vi "Example.vi"   [LabVIEW 2018]
uses:
  src/MPU.lvclass
  <vilib>/rvi/DataTransferAndStorage/Container/Common/niFpgaContainerGetUniqueNameForEmu.vi
  <vilib>/rvi/DataTransferAndStorage/Container/Common/niFpgaContainerSetEmuInfo.vi
  <vilib>/rvi/eio/common/nirviEmuReportErrorAndStop.vi
  <vilib>/rvi/LocalResourceManager/LocalResourceManager.xnode
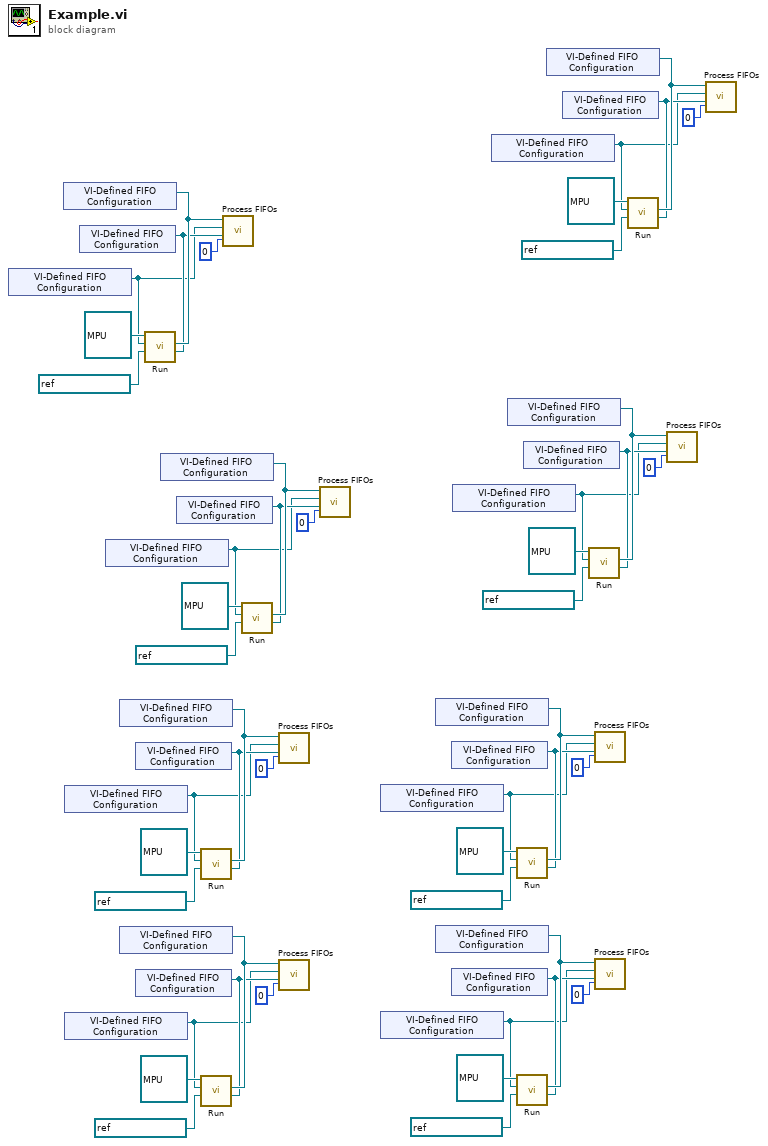
[diagram p0: block diagram]
diagram:
  n1 = xnode "VI-Defined FIFO Configuration"() -> ("FIFO Out"=w43:refnum<k21>)
  n2 = xnode "VI-Defined FIFO Configuration"() -> ("FIFO Out"=w46:refnum<k21>)
  n3 = xnode "VI-Defined FIFO Configuration"() -> ("FIFO Out"=w19:refnum<k21>)
  n4 = xnode "VI-Defined FIFO Configuration"() -> ("FIFO Out"=w7:refnum<k21>)
  n5 = xnode "VI-Defined FIFO Configuration"() -> ("FIFO Out"=w45:refnum<k21>)
  n6 = xnode "VI-Defined FIFO Configuration"() -> ("FIFO Out"=w31:refnum<k21>)
  n7 = xnode "VI-Defined FIFO Configuration"() -> ("FIFO Out"=w22:refnum<k21>)
  n8 = xnode "VI-Defined FIFO Configuration"() -> ("FIFO Out"=w10:refnum<k21>)
  n9 = xnode "VI-Defined FIFO Configuration"() -> ("FIFO Out"=w21:refnum<k21>)
  n10 = xnode "VI-Defined FIFO Configuration"() -> ("FIFO Out"=w9:refnum<k21>)
  n11 = call-dynamic "Run.vi"("DebugOut"=w45, "Telemetry"=w46, "Port"=refnum<k21> "Mod1\\Port1", "Command FIFO"=w43, "MPU in"=refnum<class "MPU.lvclass"> refnum ("Modbus_Processing_Unit.lvlib:MPU.lvclass")) -> ()  [unwired: 4 in, 2 out]
  n12 = xnode "VI-Defined FIFO Configuration"() -> ("FIFO Out"=w34:refnum<k21>)
  n13 = xnode "VI-Defined FIFO Configuration"() -> ("FIFO Out"=w33:refnum<k21>)
  n14 = call-dynamic "Run.vi"("DebugOut"=w21, "Telemetry"=w22, "Port"=refnum<k21> "Mod1\\Port3", "Command FIFO"=w19, "MPU in"=refnum<class "MPU.lvclass"> refnum ("Modbus_Processing_Unit.lvlib:MPU.lvclass")) -> ()  [unwired: 4 in, 2 out]
  n15 = call-dynamic "Run.vi"("DebugOut"=w9, "Telemetry"=w10, "Port"=refnum<k21> "Mod1\\Port4", "Command FIFO"=w7, "MPU in"=refnum<class "MPU.lvclass"> refnum ("Modbus_Processing_Unit.lvlib:MPU.lvclass")) -> ()  [unwired: 4 in, 2 out]
  n16 = call "Process FIFOs.vi"("Timeout"=0, "FIFO Out 2"=w45, "FIFO Out"=w43, "Refnum in"=w46) -> ()  [unwired: 7 in, 1 out]
  n17 = call-dynamic "Run.vi"("DebugOut"=w33, "Telemetry"=w34, "Port"=refnum<k21> "Mod1\\Port2", "Command FIFO"=w31, "MPU in"=refnum<class "MPU.lvclass"> refnum ("Modbus_Processing_Unit.lvlib:MPU.lvclass")) -> ()  [unwired: 4 in, 2 out]
  n18 = call "Process FIFOs.vi"("Timeout"=0, "FIFO Out 2"=w21, "FIFO Out"=w19, "Refnum in"=w22) -> ()  [unwired: 7 in, 1 out]
  n19 = call "Process FIFOs.vi"("Timeout"=0, "FIFO Out 2"=w9, "FIFO Out"=w7, "Refnum in"=w10) -> ()  [unwired: 7 in, 1 out]
  n20 = call "Process FIFOs.vi"("Timeout"=0, "FIFO Out 2"=w33, "FIFO Out"=w31, "Refnum in"=w34) -> ()  [unwired: 7 in, 1 out]
  n21 = xnode "VI-Defined FIFO Configuration"() -> ("FIFO Out"=w13:refnum<k21>)
  n22 = xnode "VI-Defined FIFO Configuration"() -> ("FIFO Out"=w1:refnum<k21>)
  n23 = xnode "VI-Defined FIFO Configuration"() -> ("FIFO Out"=w16:refnum<k21>)
  n24 = xnode "VI-Defined FIFO Configuration"() -> ("FIFO Out"=w4:refnum<k21>)
  n25 = xnode "VI-Defined FIFO Configuration"() -> ("FIFO Out"=w15:refnum<k21>)
  n26 = xnode "VI-Defined FIFO Configuration"() -> ("FIFO Out"=w3:refnum<k21>)
  n27 = xnode "VI-Defined FIFO Configuration"() -> ("FIFO Out"=w25:refnum<k21>)
  n28 = xnode "VI-Defined FIFO Configuration"() -> ("FIFO Out"=w37:refnum<k21>)
  n29 = xnode "VI-Defined FIFO Configuration"() -> ("FIFO Out"=w28:refnum<k21>)
  n30 = call-dynamic "Run.vi"("DebugOut"=w15, "Telemetry"=w16, "Port"=refnum<k21> "Mod2\\Port3", "Command FIFO"=w13, "MPU in"=refnum<class "MPU.lvclass"> refnum ("Modbus_Processing_Unit.lvlib:MPU.lvclass")) -> ()  [unwired: 4 in, 2 out]
  n31 = call-dynamic "Run.vi"("DebugOut"=w3, "Telemetry"=w4, "Port"=refnum<k21> "Mod2\\Port4", "Command FIFO"=w1, "MPU in"=refnum<class "MPU.lvclass"> refnum ("Modbus_Processing_Unit.lvlib:MPU.lvclass")) -> ()  [unwired: 4 in, 2 out]
  n32 = xnode "VI-Defined FIFO Configuration"() -> ("FIFO Out"=w27:refnum<k21>)
  n33 = xnode "VI-Defined FIFO Configuration"() -> ("FIFO Out"=w40:refnum<k21>)
  n34 = xnode "VI-Defined FIFO Configuration"() -> ("FIFO Out"=w39:refnum<k21>)
  n35 = call-dynamic "Run.vi"("DebugOut"=w27, "Telemetry"=w28, "Port"=refnum<k21> "Mod2\\Port2", "Command FIFO"=w25, "MPU in"=refnum<class "MPU.lvclass"> refnum ("Modbus_Processing_Unit.lvlib:MPU.lvclass")) -> ()  [unwired: 4 in, 2 out]
  n36 = call "Process FIFOs.vi"("Timeout"=0, "FIFO Out 2"=w15, "FIFO Out"=w13, "Refnum in"=w16) -> ()  [unwired: 7 in, 1 out]
  n37 = call "Process FIFOs.vi"("Timeout"=0, "FIFO Out 2"=w3, "FIFO Out"=w1, "Refnum in"=w4) -> ()  [unwired: 7 in, 1 out]
  n38 = call-dynamic "Run.vi"("DebugOut"=w39, "Telemetry"=w40, "Port"=refnum<k21> "Mod2\\Port1", "Command FIFO"=w37, "MPU in"=refnum<class "MPU.lvclass"> refnum ("Modbus_Processing_Unit.lvlib:MPU.lvclass")) -> ()  [unwired: 4 in, 2 out]
  n39 = call "Process FIFOs.vi"("Timeout"=0, "FIFO Out 2"=w27, "FIFO Out"=w25, "Refnum in"=w28) -> ()  [unwired: 7 in, 1 out]
  n40 = call "Process FIFOs.vi"("Timeout"=0, "FIFO Out 2"=w39, "FIFO Out"=w37, "Refnum in"=w40) -> ()  [unwired: 7 in, 1 out]
